vi "saveDistributionToFile.vi"(8 "2D data":dbl[][](array[numeric]) format="%0.2f", 9 "Camera calibration factor (mm/px)":dbl, 10 "yi":dbl, 11 "file path (use dialog)":path) -> (3 "Header text":string)   [LabVIEW 2014]
uses:
  <vilib>/Utility/file.llb/Write To Spreadsheet File (DBL).vi
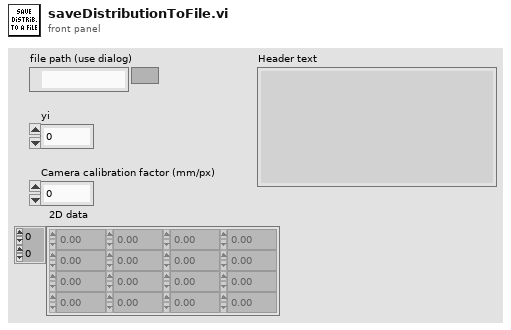
[diagram p1: front panel]
types:
  T1 = enum16{"open", "replace", "create", "open or create", "replace or create", "replace or create with confirmation"}
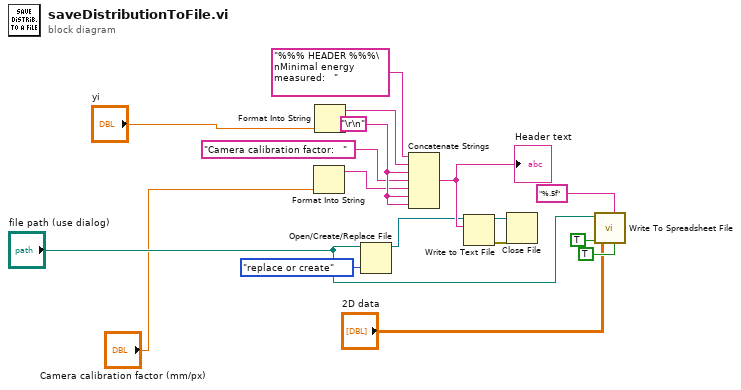
[diagram p0: block diagram]
diagram:
  w8 = "\r\n"
  n1 = Format Into String("Camera calibration factor (mm/px)") -> (resulting string=w6:string)  [unwired: 3 in, 1 out]
  n2 = Format Into String("yi") -> (resulting string=w3:string)  [unwired: 3 in, 1 out]
  n3 = Open/Create/Replace File(file path (use dialog)="file path (use dialog)", operation (0:open)=T1."replace or create") -> (refnum out=w9:refnum<file>)  [unwired: 4 in, 2 out]
  n4 = Concatenate Strings("%%% HEADER %%%\nMinimal energy measured:   " ("string"), w3, w8, "Camera calibration factor:   " ("string"), w6, w8, w8) -> (w10:string)
  "Header text" <- w10
  n5 = Write to Text File(file (use dialog)=w9, text=w10) -> (refnum out=w17:refnum<file>, error out=w16:errorcluster)  [unwired: 2 in, 1 out]
  n6 = Close File(refnum=w17, error in=w16) -> ()  [unwired: 2 out]
  n7 = call-poly <vilib>:"Write To Spreadsheet File.vi"("transpose? (no:F)"=TRUE, "format (%.3f)"="%.5f", "append to file? (new file:F)"=TRUE, "2D data"="2D data", "file path (dialog if empty)"="file path (use dialog)") -> ()  [unwired: 3 in, 1 out]
